vi "statuptest.vi"() -> ()   [LabVIEW 2018]
uses:
  <vilib>/Platform/TimedLoop/XDataNode/timing_clust.ctl
  <vilib>/Platform/TimedLoop/XDataNode/nitl_modes.ctl
  <vilib>/Platform/TimedLoop/XDataNode/wakeup.ctl
  <vilib>/platform/TimedLoop/XDataNode/XDataNode.xnode
  <vilib>/Platform/TimedLoop/XDataNode/XDNodeRunTimeDep.lvlib
panel:
  out "appended array":dbl[](array[numeric])
  in  "Stop Button":bool
  out "Data buffer":dbl[](array[numeric])
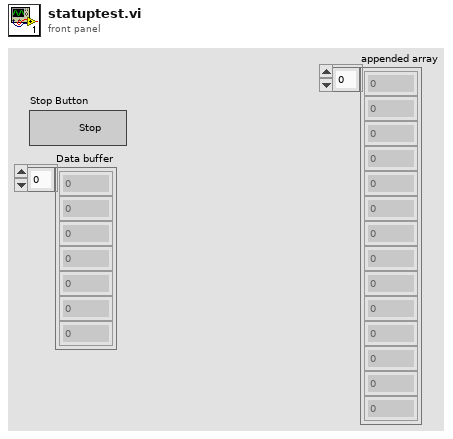
[diagram p1: front panel]
types:
  T1 = typedef "XDNodeRunTimeDep.lvlib/timing_clust.ctl" = cluster{"Expected End [f-1]":u64, "Actual End [f-1]":u64, "Finished Late? [f-1]":bool, "Expected End [i-1]":u64, "Actual End [i-1]":u64, "Finished Late? [i-1]":bool, "Expected Start [i]":u64, "Actual Start [i]":u64, "Expected Start [f]":u64, "Actual Start [f]":u64, "Source Name":string, "Structure Name":string, "Period":i64, "Deadline":i64, "Offset":i64, "Start":i64, "Priority":i32, "Timeout":i32, "Mode":T2, "Wakeup Reason":T3, "Error":errorcluster, "Source Type":string, "Secondary Source Type":string, "Global End Time":u64, "Global Start Time":u64, "Frame Duration":u64, "Iteration Duration":u64, "Assigned CPU":i32, "I/O Scan Engine Mode":u32}
  T2 = typedef "XDNodeRunTimeDep.lvlib/nitl_modes.ctl" = enum32{"No Change", "Process missed periods, maintain original phase", "Discard missed periods, maintain original phase", "Process missed periods, ignore original phase", "Discard missed periods, ignore original phase"}
  T3 = typedef "XDNodeRunTimeDep.lvlib/wakeup.ctl" = enum32{"Normal", "Aborted", "Asynchronous wakeup", "Timing source error", "Timed loop error", "Timeout"}
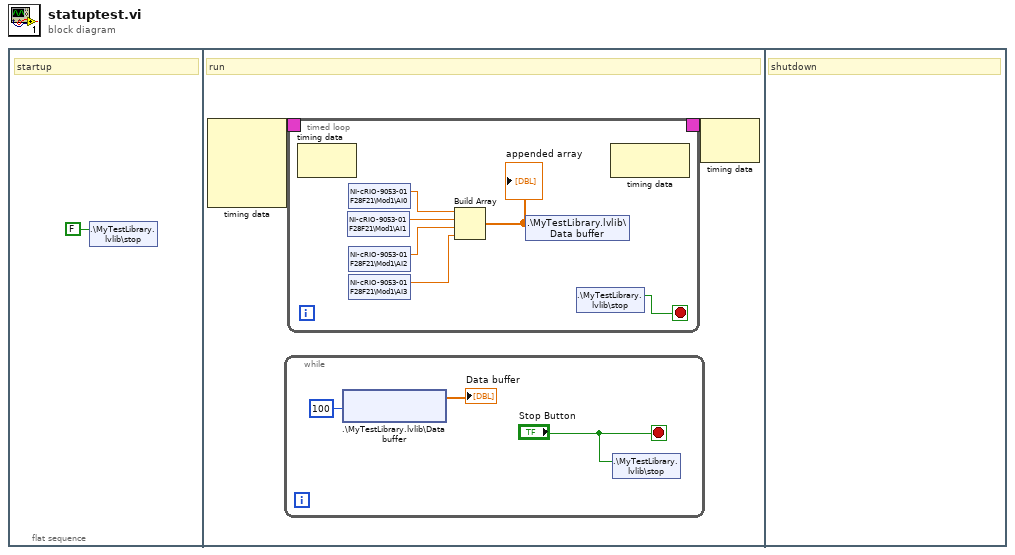
[diagram p0: block diagram]
diagram:
  n1 = flat-sequence {
    frame #0 {
      # "startup"
      n2 = shared-variable ".\\MyTestLibrary.lvlib\\stop"(FALSE ("stop")) -> ()  [unwired: 1 in, 1 out]
    }
    frame #1 {
      # "run"
      n3 = node-c288() -> (w3:T1)  [unwired: 4 in]
      n4 = while {
        stop <- "Stop Button" stop-if-true
        n5 = shared-variable ".\\MyTestLibrary.lvlib\\Data buffer"(100 ("ms timeout (0)")) -> (→"Data buffer":dbl[])  [unwired: 1 in, 2 out]
        n6 = shared-variable ".\\MyTestLibrary.lvlib\\stop"("Stop Button") -> ()  [unwired: 1 in, 1 out]
      }
      n7 = timed-loop {
        timing: w3 -> [_]
        timing-out: [_] -> w2
        stop <- w7 stop-if-true
        n8 = node-c288() -> ()  [unwired: 1 in, 1 out]
        n9 = shared-variable "NI-cRIO-9053-01F28F21\\Mod1\\AI1"() -> (w11:dbl)  [unwired: 1 in, 1 out]
        n10 = shared-variable "NI-cRIO-9053-01F28F21\\Mod1\\AI0"() -> (w12:dbl)  [unwired: 1 in, 1 out]
        n11 = shared-variable "NI-cRIO-9053-01F28F21\\Mod1\\AI2"() -> (w10:dbl)  [unwired: 1 in, 1 out]
        n12 = shared-variable "NI-cRIO-9053-01F28F21\\Mod1\\AI3"() -> (w9:dbl)  [unwired: 1 in, 1 out]
        n13 = Build Array(w12, w11, w10, w9) -> (w8:dbl[])
        "appended array" <- w8
        n14 = shared-variable ".\\MyTestLibrary.lvlib\\Data buffer"(w8) -> ()  [unwired: 1 in, 1 out]
        n15 = shared-variable ".\\MyTestLibrary.lvlib\\stop"() -> (w7:bool)  [unwired: 1 in, 1 out]
        n16 = node-c288() -> ()  [unwired: 1 in, 1 out]
      }
      n17 = node-c288(w2) -> ()  [unwired: 1 out]
    }
    frame #2 {
      # "shutdown"
    }
  }
